vi "Volume acq videos-Initialise.vi"(8 "error in (no error)":errorcluster, 10 "Channel":T3, 11 "created path":path) -> (0 "error out":errorcluster, 2 "Temp Image":T1, 3 "Refnum out":T2)   [LabVIEW 2017]
uses:
  Typedefs/Channel Selector.ctl
  <vilib>/vision/Avi.llb/IMAQ AVI2 Refnum.ctl
  <vilib>/vision/Image Controls.llb/IMAQ Image.ctl
panel:
  # "RE-ENTRANT"
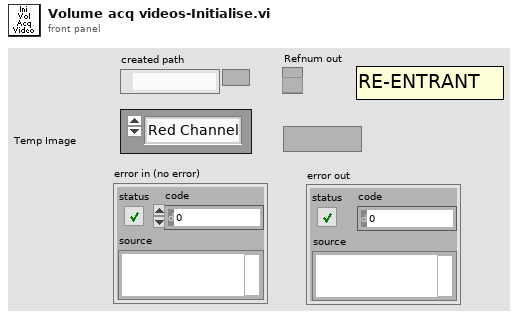
[diagram p1: front panel]
types:
  T1 = typedef "IMAQ Image.ctl" = refnum<image>
  T2 = typedef "IMAQ AVI2 Refnum.ctl" = refnum<k20>
  T3 = typedef "Channel Selector.ctl" = enum16{"Red Channel", "Green Channel", "Blended"}
  T4 = typedef "Image Type" = u32
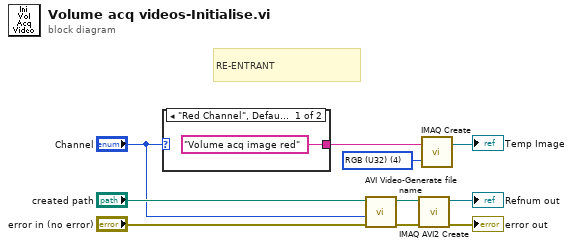
[diagram p0: block diagram]
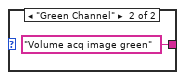
[diagram p2: hidden frame]
diagram:
  w3 = T4 4 items=["Grayscale (U8)", "Grayscale (I16)", "Grayscale (SGL)", "Complex (CSG)", "RGB (U32)", "HSL (U32)", "RGB (U64)", "Grayscale (U16)"] ("Image Type")
  # "RE-ENTRANT"
  n1 = case shown="\"Red Channel\", Default" "Channel" {
    tunnel: ["Volume acq image red" ("Image Name") "Volume acq image green" ("Image Name")] -> w2
    frame "Red Channel", Default {
    }
    frame "Green Channel" {
    }
  }
  n2 = call "AVI Video-Generate file name.vi"("error in (no error)"="error in (no error)", "Channel"="Channel", "Videos folder path"="created path") -> ("error out"=w7:errorcluster, "AVI file path & name"=w6:path)  [unwired: 7 in]
  n3 = call "IMAQ AVI2 Create"("error in (no error)"=w7, "AVI Path"=w6) -> ("error out"=→"error out":errorcluster, "AVI Refnum"=→"Refnum out":T2)  [unwired: 8 in]
  n4 = call "IMAQ Create"("Image Name"=w2, "Image Type"=w3) -> ("New Image"=→"Temp Image":T1)  [unwired: 2 in, 2 out]
